vi "ConfigureOutput.vi"(8 "error in (no error)":errorcluster, 10 "Output((F)":bool, 11 "YP03-60_Y in":refnum<class "YP03-60_Y.lvclass">) -> (0 "error out":errorcluster, 3 "YP03-60_Y out":refnum<class "YP03-60_Y.lvclass">)   [LabVIEW 2020, in "PowerControl.lvlib" / "YP03-60_Y.lvclass"]
uses:
  YP03-60_Y.lvclass
  YP03-60_Y.lvclass/YP03-60_Y.ctl
  <vilib>/Instr/_visa.llb/VISA Configure Serial Port (Instr).vi
  YP03-60_X/YP03-60_X.lvclass
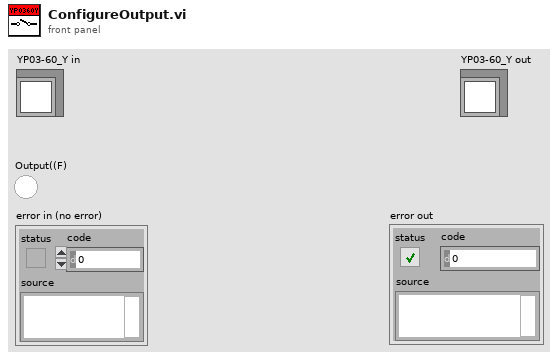
[diagram p1: front panel]
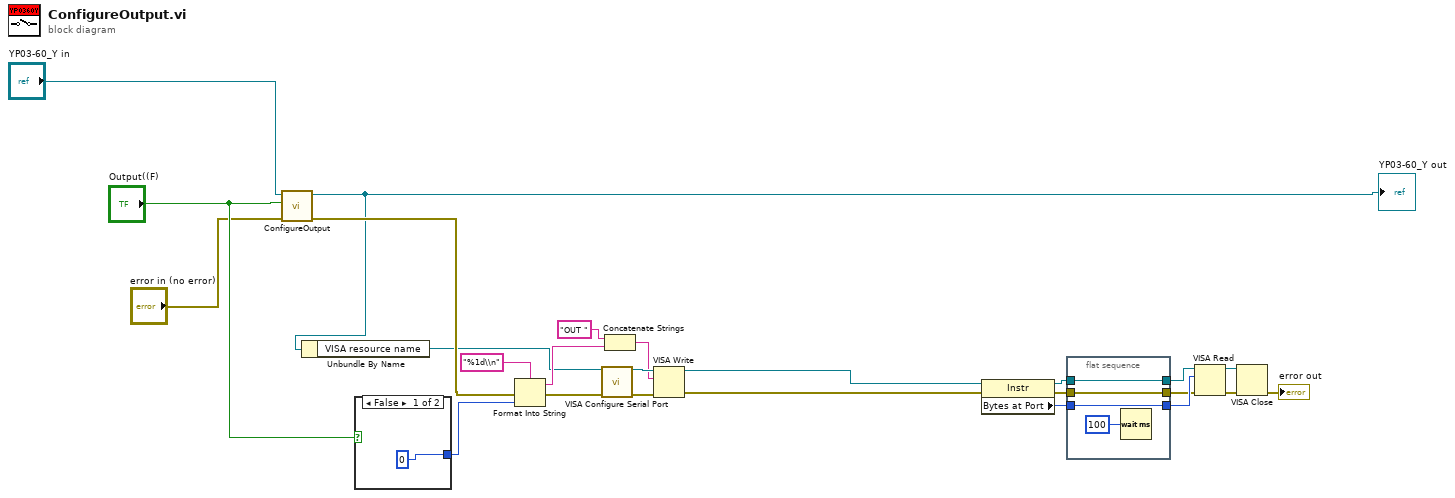
[diagram p0: block diagram]
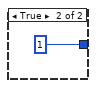
[diagram p2: hidden frame]
diagram:
  n1 = call-parent "ConfigureOutput.vi"("error in (no error)"="error in (no error)", "Output((F)"="Output((F)", "YP03-60_X in"="YP03-60_Y in") -> ("error out 2"=w17:errorcluster, "YP03-60_X out"=w2:refnum<class "YP03-60_Y.lvclass">)  [unwired: 7 in]
  "YP03-60_Y out" <- w2
  n2 = Unbundle By Name(w2) -> ("VISA resource name"=w1:refnum<visa-resource-name>)
  n3 = case shown="False" "Output((F)" {
    tunnel: [0 1] -> w25
    frame False {
    }
    frame True {
    }
  }
  n4 = Format Into String(format string="%1d\\n", error in=w17, w25) -> (resulting string=w14:string, error out=w19:errorcluster)  [unwired: 1 in]
  n5 = call-poly "VISA Configure Serial Port"("VISA resource name"=w1, "error in (no error)"=w19) -> ("VISA resource name out"=w21:refnum<visa-resource-name>, "error out"=w20:errorcluster)  [unwired: 12 in]
  n6 = Concatenate Strings("OUT " ("string"), w14) -> (w11:string)
  n7 = VISA Write(VISA resource name=w21, write buffer=w11, error in (no error)=w20) -> (VISA resource name out=w13:refnum<visa-resource-name>, error out=w12:errorcluster)  [unwired: 1 out]
  n8 = property class="Instr"(reference=w13, error in=w12) -> (reference out=w8:refnum<visa-resource-name>, error out=w6:errorcluster, "Bytes at Port"=w10:u32)
  n9 = flat-sequence {
    tunnel: w8 -> [w31]
    tunnel: [w31] -> w7
    tunnel: [w30] -> w5
    tunnel: w6 -> [w30]
    tunnel: [w29] -> w9
    tunnel: w10 -> [w29]
    frame #0 {
      n10 = Wait (ms)(milliseconds to wait=u32 100) -> ()  [unwired: 1 out]
    }
  }
  n11 = VISA Read(VISA resource name=w7, byte count=w9, error in (no error)=w5) -> (VISA resource name out=w24:refnum<visa-resource-name>, error out=w22:errorcluster)  [unwired: 2 out]
  n12 = VISA Close(VISA resource name=w24, error in (no error)=w22) -> (error out=→"error out":errorcluster)
